vi "ecuacion_simulacion_en_el_tiempo.vi"(0 "set point":dbl, 1 "e(k-1)":dbl, 2 "e(k-2)":dbl, 5 "yk":dbl, 7 "q0":dbl, 9 "q1":dbl, 11 "q2":dbl, 12 "u(k-1)":dbl) -> (4 "e(k-1) actualizado":dbl, 15 "u(k)":dbl)   [LabVIEW 2020]
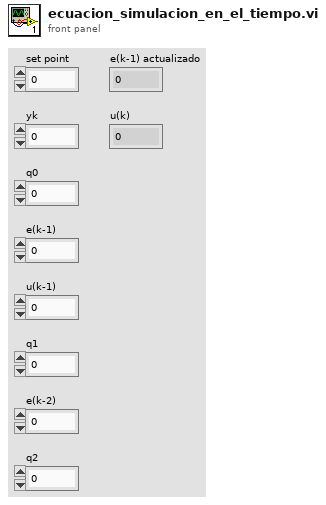
[diagram p1: front panel]
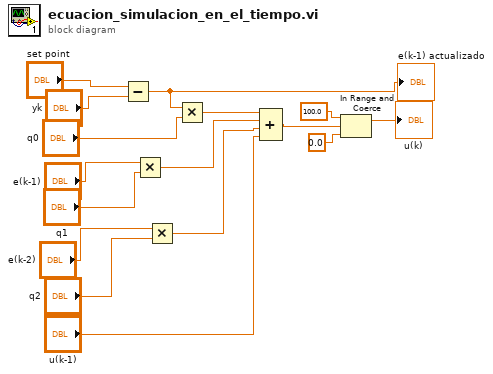
[diagram p0: block diagram]
diagram:
  n1 = Subtract(x="set point", y="yk") -> (x-y=w15:dbl)
  "e(k-1) actualizado" <- w15
  n2 = Multiply(x="e(k-1)", y="q1") -> (x*y=w7:dbl)
  n3 = Multiply(x="e(k-2)", y="q2") -> (x*y=w10:dbl)
  n4 = Multiply(x=w15, y="q0") -> (x*y=w4:dbl)
  n5 = Compound Arithmetic op=ADD(w4, w7, w10, "u(k-1)") -> (w14:dbl)
  n6 = In Range and Coerce(upper limit=100.0, x=w14, lower limit=0.0) -> (coerced(x)=→"u(k)":dbl)  [unwired: 1 out]
